vi "Create Group Section Only.vi"(8 "error in (no error)":errorcluster, 9 "String":string, 10 "dsf refnum in":refnum<class "Configuration Session.lvclass">, 11 "Section Ptr":T1 format="%.0x") -> (0 "error out":errorcluster)   [LabVIEW 2017, in "DSF System Explorer.lvlib"]
uses:
  DSF System Explorer.lvlib
  <vilib>/NI Veristand/Custom Device API/Custom Device Item Ref.ctl
  DSF Core.lvlibp/Classes/Configuration/Configuration Session.lvclass
  DSF Core.lvlibp/Classes/Configuration/Read Plugin Group IDs.vi
  Shared/Group Page GUID.vi
  <vilib>/NI Veristand/Custom Device API/Set Item Property (String).vi
  <vilib>/NI Veristand/Custom Device API/Custom Device API.lvlib
  Shared/DSF Shared.lvlib
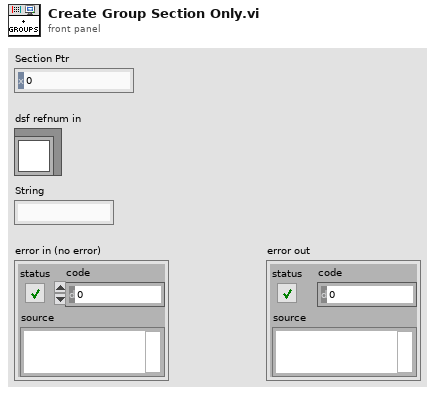
[diagram p1: front panel]
types:
  T1 = typedef "Custom Device API.lvlib/Custom Device Item Ref.ctl" = u64
  T2 = typedef "DSF System Explorer.lvlib/shared data ref.ctl" = refnum<data-value>
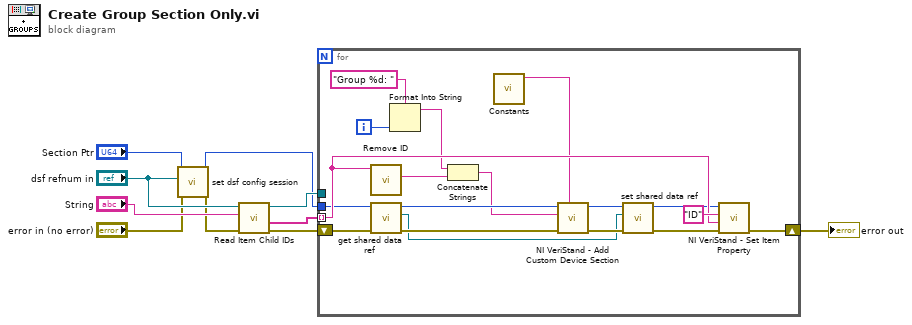
[diagram p0: block diagram]
diagram:
  n1 = call "set dsf config session.vi"("error in (no error)"="error in (no error)", "Configuration Session"="dsf refnum in", "Item Ref in"="Section Ptr") -> ("error out"=w2:errorcluster, "Item Ref out"=w4:T1)  [unwired: 7 in]
  n2 = call-poly "Read Item Child IDs.vi"("error in (no error)"=w2, "Plugin ID"="String", "Configuration Session"="dsf refnum in") -> ("error out"=w9:errorcluster, "Group IDs"=w8:string[], "Configuration Session out"=w7:refnum<class "Configuration Session.lvclass">)  [unwired: 5 in, 1 out]
  n3 = for {
    tunnel: w8 -> [w27] mode=indexing
    tunnel: w4 -> [w26]
    tunnel: w7 -> [_]
    shift-right: [w12] -> w1
    shift-left: w9 -> [w25]
    i -> [w16]
    n4 = call "Remove ID.vi"("id string"=w27) -> ("name"=w15:string)  [unwired: 8 in, 2 out]
    n5 = call "get shared data ref.vi"("error in (no error)"=w25, "Item Ref in"=w26) -> ("error out"=w24:errorcluster, "shared data ref"=w18:T2, "Item Ref out"=w23:T1)  [unwired: 7 in]
    n6 = Format Into String(format string="Group %d: ", w16) -> (resulting string=w14:string)  [unwired: 2 in, 1 out]
    n7 = Concatenate Strings(w14, w15) -> (w13:string)
    n8 = call-poly "Constants.vi"() -> ("Group GUID"=w17:string)  [unwired: 11 in]
    n9 = call <vilib>:"NI VeriStand - Add Custom Device Section.vi"("GUID (Default Section)"=w17, "error in (no error)"=w24, "Section Name"=w13, "Parent Ref in"=w23) -> ("error out"=w22:errorcluster, "Section Ptr"=w21:T1)  [unwired: 4 in, 2 out]
    n10 = call "set shared data ref.vi"("error in (no error)"=w22, "shared data ref"=w18, "Node Ptr"=w21) -> ("error out"=w19:errorcluster, "Item Ref out"=w20:T1)  [unwired: 7 in]
    n11 = call-poly <vilib>:"NI VeriStand - Set Item Property.vi"("error in (no error)"=w19, "Value"=w27, "Property Name"="ID", "Item Ref in"=w20) -> ("error out"=w12:errorcluster)  [unwired: 5 in, 2 out]
  }
  "error out" <- w1
